vi "FTW-JSON-Unescape.vi"(1 "Escaped UTF-8 String":string) -> (0 "Unescaped String":string)   [LabVIEW 2014]
panel:
  # "Inputs"
  # "Outputs"
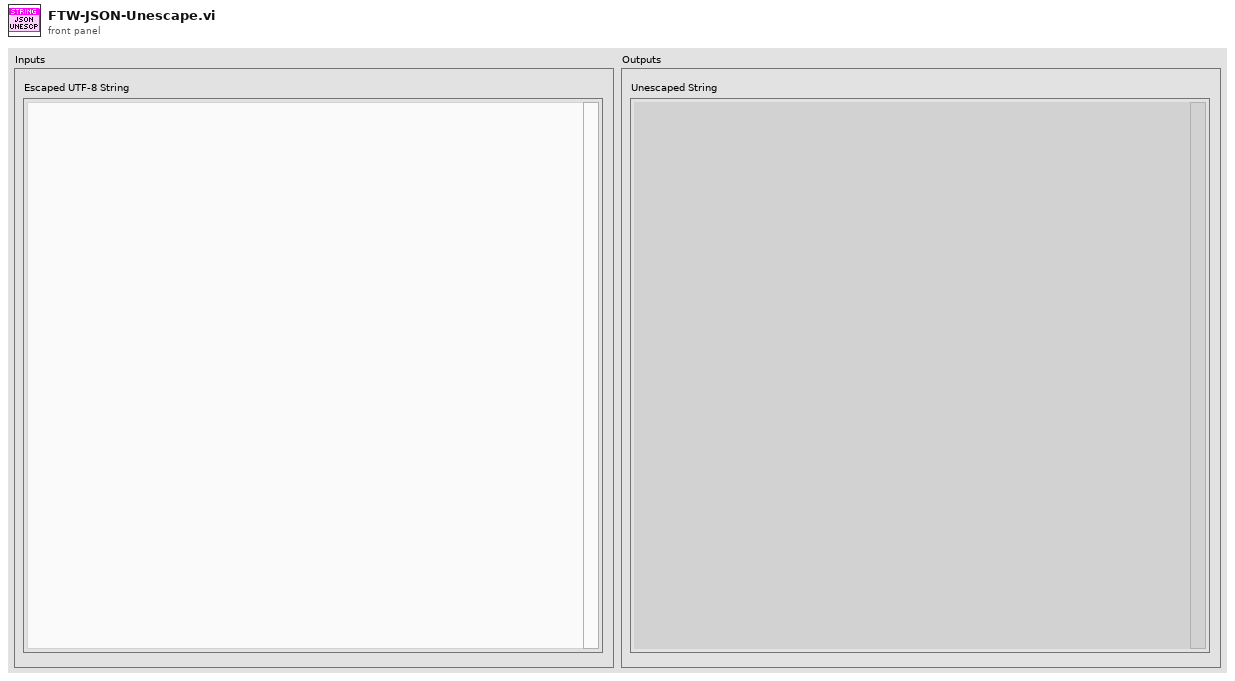
[diagram p1: front panel]
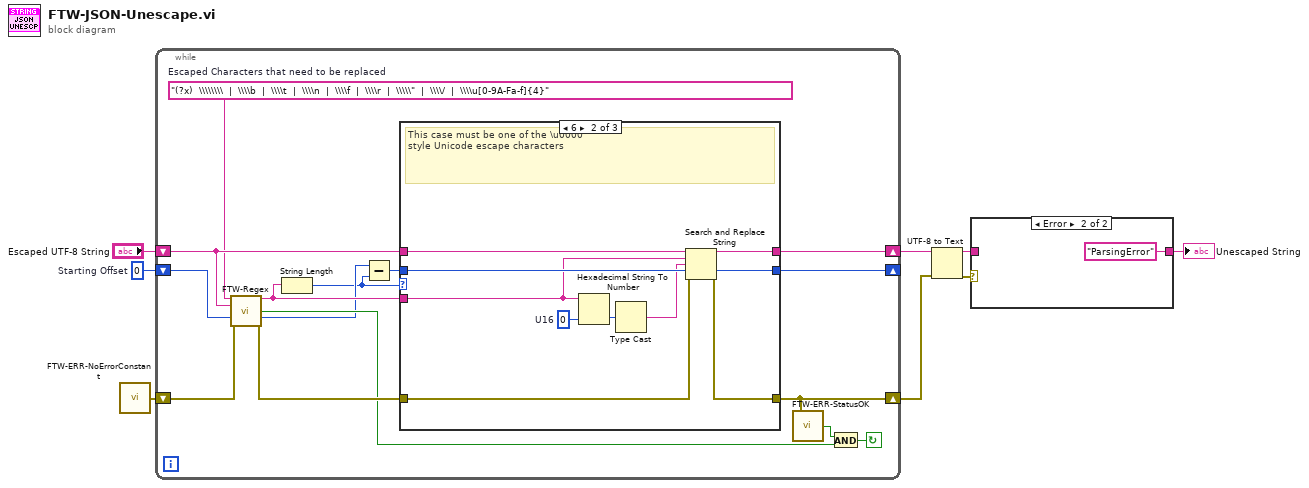
[diagram p0: block diagram]
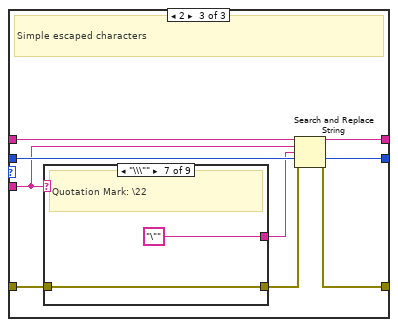
[diagram p3: hidden frame]
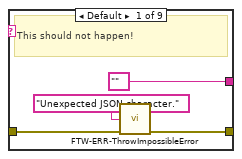
[diagram p4: hidden frame]
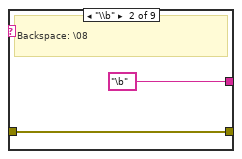
[diagram p5: hidden frame]
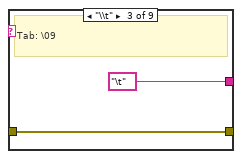
[diagram p6: hidden frame]
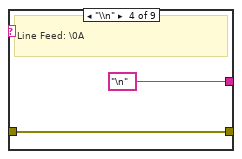
[diagram p7: hidden frame]
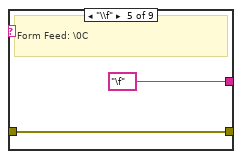
[diagram p8: hidden frame]
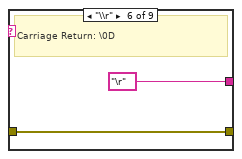
[diagram p9: hidden frame]
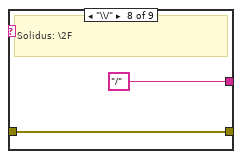
[diagram p10: hidden frame]
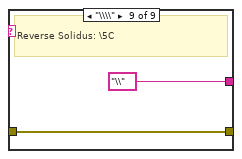
[diagram p11: hidden frame]
diagram:
  w3 = 0  # Starting Offset
  n1 = call "FTW-ERR-NoErrorConstant.vi"() -> ("no error"=w8:errorcluster)
  n2 = while {
    shift-right: [w21] -> w2
    shift-left: "Escaped UTF-8 String" -> [w22]
    shift-right: [w16] -> w1
    shift-left: w8 -> [w23]
    shift-right: [w14] -> _
    shift-left: w3 -> [w19]
    stop <- w17 continue-if-true
    w12 = "(?x)  \\\\\\\\  |  \\\\b  |  \\\\t  |  \\\\n  |  \\\\f  |  \\\\r  |  \\\\\"  |  \\\\/  |  \\\\u[0-9A-Fa-f]{4}"  # Escaped Characters that need to be replaced
    n3 = call "FTW-Regex.vi"("Regular Expression"=w12, "Input String"=w22, "Starting Offset"=w19, "error in"=w23) -> ("Match"=w13:string, "Match Found?"=w18:bool, "Offset after Match"=w11:i32, "error out"=w20:errorcluster)  [unwired: 7 in, 1 out]
    n4 = String Length(string=w13) -> (length=w9:i32)
    n5 = Subtract(x=w11, y=w9) -> (x-y=w10:i32)
    n6 = case shown="6" w9 {
      tunnel: w22 -> [w25 w35 w44]
      tunnel: [w25 w34 w43] -> w21
      tunnel: [w26 w32 w42] -> w16
      tunnel: w20 -> [w26 w33 w40]
      tunnel: [w24 w31 w41] -> w14
      tunnel: w10 -> [w24 w36 w45]
      tunnel: w13 -> [_ w30 w38]
      frame Default {
        # "Empty match signals we're finished"
      }
      frame 6 {
        w29 = u32 0  # U16
        # "This case must be one of the \\u0000\nstyle Unicode escape characters"
        n7 = Hexadecimal String To Number(string=w30, default (0uL)=w29) -> (number=w28:u32)  [unwired: 1 in, 1 out]
        n8 = Type Cast(x=w28) -> (*(type *) &x=w27:string)  [unwired: 1 in]
        n9 = Search and Replace String(input string=w35, search string=w30, replace string=w27, offset=w36, error in=w33) -> (result string=w34:string, offset past replacement=w31:i32, error out=w32:errorcluster)  [unwired: 3 in, 1 out]
      }
      frame 2 {
        # "Simple escaped characters"
        n10 = case shown="\"\\\\\\\"\"" w38 {
          tunnel: ["" "\b" "\t" "\n" "\f" "\r" "\"" "/" "\\"] -> w37
          tunnel: w40 -> [w48 w50 w52 w54 w56 w58 w60 w62 w64]
          tunnel: [w47 w50 w52 w54 w56 w58 w60 w62 w64] -> w39
          frame Default {
            # "This should not happen!"
            n11 = call "FTW-ERR-ThrowImpossibleError.vi"("Reason this error should never happen"="Unexpected JSON character.", "error in"=w48) -> ("error out"=w47:errorcluster)  [unwired: 13 in]
          }
          frame "\\b" {
            # "Backspace: \\08"
          }
          frame "\\t" {
            # "Tab: \\09"
          }
          frame "\\n" {
            # "Line Feed: \\0A"
          }
          frame "\\f" {
            # "Form Feed: \\0C"
          }
          frame "\\r" {
            # "Carriage Return: \\0D"
          }
          frame "\\\"" {
            # "Quotation Mark: \\22"
          }
          frame "\\/" {
            # "Solidus: \\2F"
          }
          frame "\\\\" {
            # "Reverse Solidus: \\5C"
          }
        }
        n12 = Search and Replace String(input string=w44, search string=w38, replace string=w37, offset=w45, error in=w39) -> (result string=w43:string, offset past replacement=w41:i32, error out=w42:errorcluster)  [unwired: 3 in, 1 out]
      }
    }
    n13 = call "FTW-ERR-StatusOK.vi"("error to check"=w16) -> ("Status OK?"=w15:bool)
    n14 = And(x=w15, y=w18) -> (x .and. y?=w17:bool)
  }
  n15 = UTF-8 to Text(8:w1, 11:w2) -> (0:w4:errorcluster, 3:w5:string)  [unwired: 1 in]
  n16 = case shown="Error" w4 {
    tunnel: [w66 "ParsingError" ("Escaped String")] -> w6
    tunnel: w5 -> [w66 _]
    frame No Error {
    }
    frame Error {
    }
  }
  "Unescaped String" <- w6
